vi "User Config Read Value.vi"(7 "Section":string, 8 "error in (no error)":errorcluster, 10 "Key":string, 11 "INI File Path":path) -> (0 "error out":errorcluster, 1 "found?":bool, 2 "Value":string, 3 "INI File Path":path)   [LabVIEW 2024]
uses:
  <vilib>/Utility/config.llb/NI_LVConfig.lvlib
  <vilib>/Utility/config.llb/Read Key (String).vi
panel:
  in  "Default":string
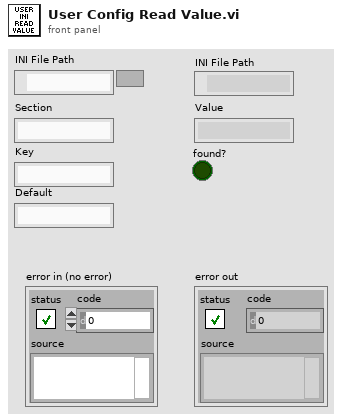
[diagram p1: front panel]
types:
  T1 = typedef "NI_LVConfig.lvlib/Config Data RefNum.ctl" = refnum<k1>
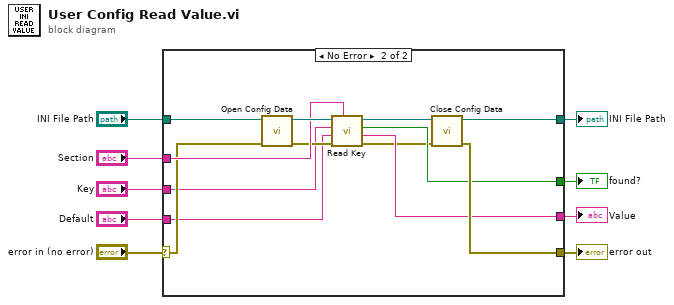
[diagram p0: block diagram]
diagram:
  n1 = case shown="No Error" "error in (no error)" {
    selector: "error in (no error)" -> [w10 w20]
    tunnel: [w10 w16] -> w8
    tunnel: "INI File Path" -> [_ w23]
    tunnel: "Section" -> [_ w21]
    tunnel: "Key" -> [_ w18]
    tunnel: [_ w15] -> w4
    tunnel: [_ w14] -> w3
    tunnel: [_ w13] -> w2
    tunnel: "Default" -> [_ w12]
    frame Error {
    }
    frame No Error {
      n2 = call <vilib>:"Open Config Data.vi"("error in (no error)"=w20, "configuration file path"=w23) -> ("error out"=w19:errorcluster, "refnum"=w22:T1)  [unwired: 7 in, 1 out]
      n3 = call-poly <vilib>:"Read Key.vi"("section"=w21, "error in (no error)"=w19, "default value"=w12, "key"=w18, "refnum"=w22) -> ("error out"=w11:errorcluster, "value"=w13:string, "found?"=w14:bool, "refnum out"=w17:T1)  [unwired: 3 in]
      n4 = call <vilib>:"Close Config Data.vi"("error in (no error)"=w11, "refnum"=w17) -> ("error out"=w16:errorcluster, "file path"=w15:path)  [unwired: 8 in]
    }
  }
  "error out" <- w8
  "Value" <- w2
  "INI File Path" <- w4
  "found?" <- w3
